vi "Find Sclera.vi"(8 "error in (no error)":errorcluster, 9 "Results":T4, 10 "Treatment":T1, 11 "Images":T2) -> (0 "error out":errorcluster, 1 "Results":T4, 2 "Treatment":T1, 3 "Images":T2)   [LabVIEW 2015]
uses:
  controls/Results.ctl
  controls/Treatment Parameters.ctl
  controls/Images.ctl
  <vilib>/vision/Image Controls.llb/IMAQ Image.ctl
  <vilib>/vision/NI_Vision_Development_Module.lvlib
panel:
  out "sclera ratio time":u32
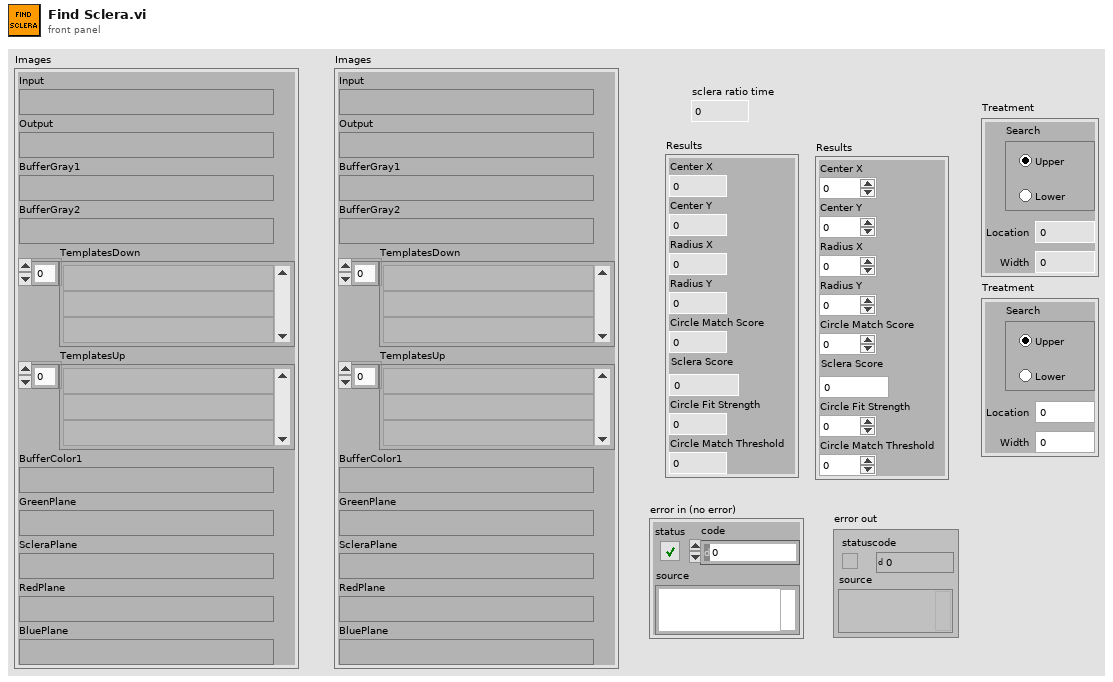
[diagram p1: front panel]
types:
  T1 = typedef "Treatment Parameters.ctl" = cluster{"Location":dbl, "Width":dbl, "Search":enum32{"Upper", "Lower"}}
  T2 = typedef "Images.ctl" = cluster{"Input":T3, "Output":T3, "BufferGray1":T3, "BufferGray2":T3, "TemplatesDown":T3[], "TemplatesUp":T3[], "BufferColor1":T3, "GreenPlane":T3, "ScleraPlane":T3, "RedPlane":T3, "BluePlane":T3}
  T3 = typedef "IMAQ Image.ctl" = refnum<image>
  T4 = typedef "Results.ctl" = cluster{"Center X":i32, "Center Y":i32, "Radius X":i32, "Radius Y":i32, "Circle Match Score":i32, "Sclera Score":dbl, "Circle Fit Strength":i32, "Circle Match Threshold":i32}
  T5 = typedef "ROI Descriptor" = cluster{"Global Rectangle":i32[], "Contours":cluster{"ID":enum32{"External", "Internal"}, "Type":u32, "Coordinates":i32[]}[]}
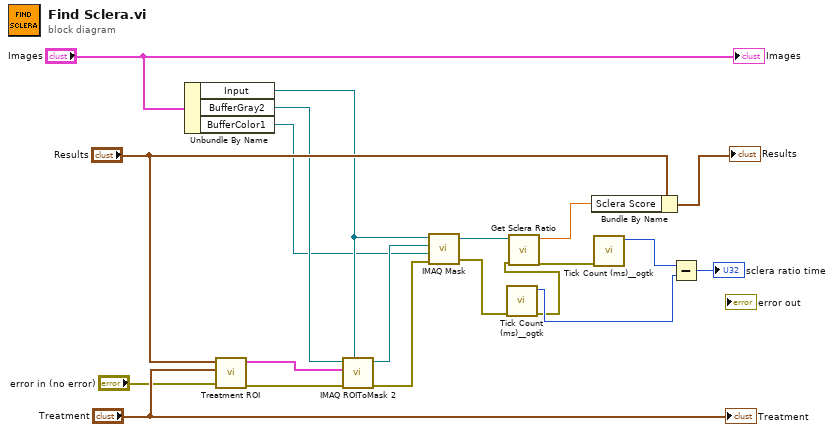
[diagram p0: block diagram]
diagram:
  n1 = Unbundle By Name("Images") -> ("Input"=w12:T3, "BufferGray2"=w10:T3, "BufferColor1"=w6:T3)
  n2 = call "Treatment ROI.vi"("error in (no error)"="error in (no error)", "Treatment"="Treatment", "Limbus"="Results") -> ("error out"=w19:errorcluster, "ROI Descriptor"=w20:T5)  [unwired: 7 in]
  n3 = call "IMAQ ROIToMask 2"("Image Model"=w12, "error in (no error)"=w19, "ROI Descriptor"=w20, "Image"=w10) -> ("error out"=w8:errorcluster, "Image Out"=w17:T3)  [unwired: 5 in, 1 out]
  n4 = call "IMAQ Mask"("error in (no error)"=w8, "Image Dst"=w6, "Image Mask"=w17, "Image Src"=w12) -> ("error out"=w7:errorcluster, "Image Dst Out"=w18:T3)  [unwired: 1 in]
  n5 = call <userlib>:"Tick Count (ms)__ogtk.vi"("error in (no error)"=w7) -> ("error out"=w3:errorcluster, "millisecond timer value"=w4:u32)  [unwired: 9 in]
  n6 = call "Get Sclera Ratio.vi"("Error In"=w3, "Image"=w18) -> ("Error Out"=w2:errorcluster, "Sclera Ratio"=w13:dbl)  [unwired: 8 in]
  n7 = Bundle By Name(cluster="Results", "Sclera Score"=w13) -> (→"Results":T4)
  n8 = call <userlib>:"Tick Count (ms)__ogtk.vi"("error in (no error)"=w2) -> ("millisecond timer value"=w1:u32)  [unwired: 9 in, 1 out]
  n9 = Subtract(x=w1, y=w4) -> (x-y=→"sclera ratio time":u32)
  "Images" <- "Images"
  "Treatment" <- "Treatment"
